vi "Encode Channels.vi"(6 "Offset":i32, 8 "error in":errorcluster, 10 "Data and Parameters":T2 {"Data" format="%.0b"}, 11 "Values in":dbl[](array[numeric])) -> (0 "error out":errorcluster, 3 "Data":u8[](array[numeric]), 4 "Number of Parameters":i32)   [LabVIEW 2020]
uses:
  <vilib>/NI/NI VeriStand Encoding and Decoding/Encoding.ctl
  b24d3698-aaae-4200-bf93-4b6af5480478.vi
  5b1080be-549e-4688-aad8-fb955257d8ef.vi
  b24d3698-aaae-4200-bf93-4b6af5480478.vi/9377bb8f-44b5-4a8f-87f1-966fd5a9edcc.vi
  b24d3698-aaae-4200-bf93-4b6af5480478.vi/e95d9d1f-307c-44d6-9f26-c3f519a4990d.vi
  b24d3698-aaae-4200-bf93-4b6af5480478.vi/0c23f515-4369-4514-bc3d-4444e6b437b2.vi
  5b1080be-549e-4688-aad8-fb955257d8ef.vi/136dcdcb-2dd3-4a4d-a796-a8f7a3f8e1ac.vi
  5b1080be-549e-4688-aad8-fb955257d8ef.vi/a54b505c-1216-4ef4-8378-3ceda9d188df.vi
  <vilib>/NI/NI VeriStand Encoding and Decoding/Get Bits Per Digit from Base.vi
  Tx UDP Execution Unit/Tx UDP Execution Unit.lvclass
  <vilib>/NI/NI VeriStand Encoding and Decoding/Encoding and Decoding.lvlib
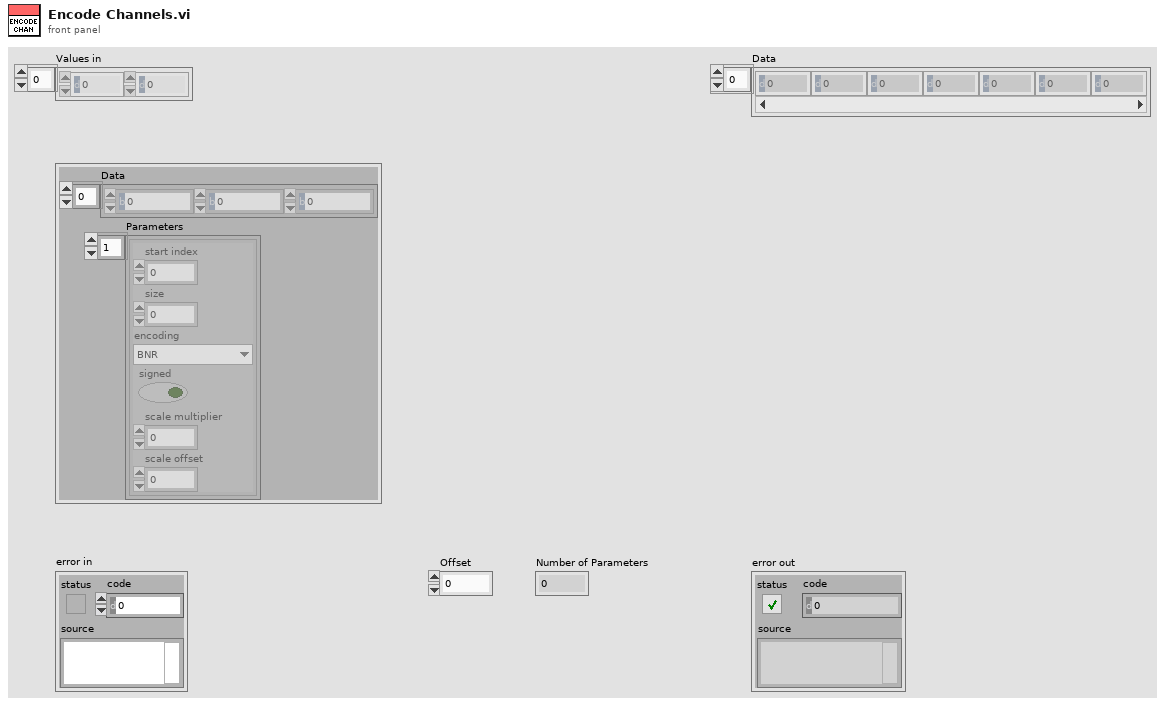
[diagram p1: front panel]
types:
  T1 = typedef "Encoding and Decoding.lvlib/Encoding.ctl" = enum16{"BNR", "BCD", "Discrete"}
  T2 = cluster{"Data":u8[], "Parameters":cluster{"start index":i32, "size":i32, "encoding":T1, "signed":bool, "scale multiplier":dbl, "scale offset":dbl}[]}
  T3 = cluster{"start index":i32, "size":i32, "encoding":T1, "signed":bool, "scale multiplier":dbl, "scale offset":dbl}[]
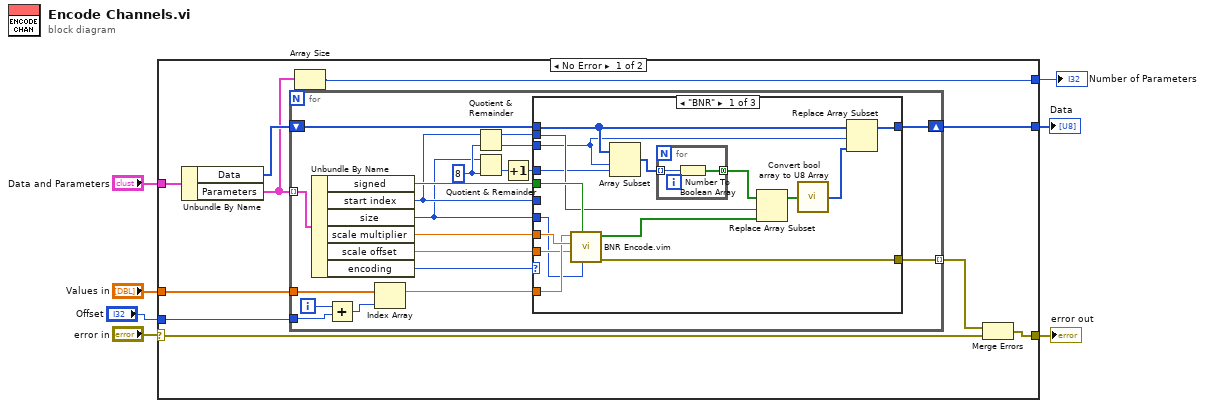
[diagram p0: block diagram]
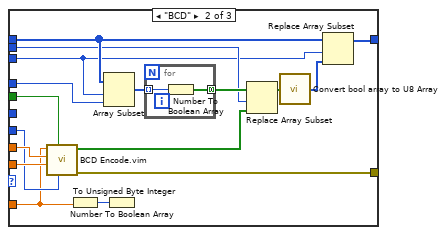
[diagram p2: hidden frame]
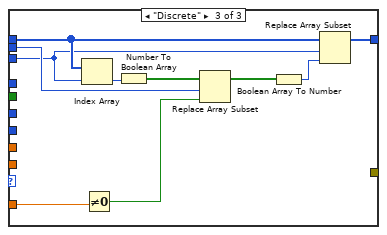
[diagram p3: hidden frame]
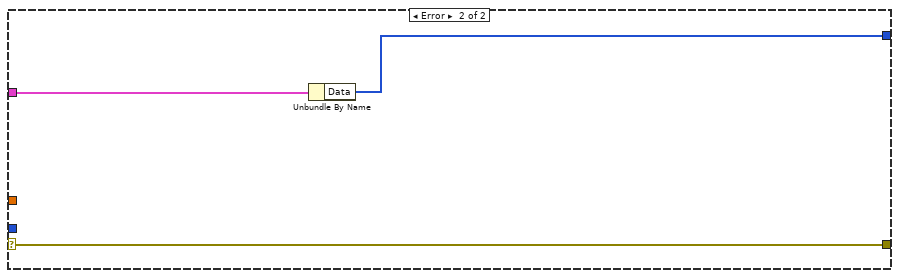
[diagram p4: hidden frame]
diagram:
  n1 = case shown="No Error" "error in" {
    selector: "error in" -> [w11 w87]
    tunnel: "Data and Parameters" -> [w17 w86]
    tunnel: "Values in" -> [w16 _]
    tunnel: [w14 w85] -> w5
    tunnel: [w12 w87] -> w3
    tunnel: "Offset" -> [w10 _]
    tunnel: [w8 _] -> w1
    frame No Error {
      n2 = Unbundle By Name(w17) -> ("Data"=w15:u8[], "Parameters"=w9:T3)
      n3 = for {
        tunnel: w16 -> [w31]
        tunnel: w9 -> [w32] mode=indexing
        shift-right: [w27] -> w14
        shift-left: w15 -> [w34]
        tunnel: [w22] -> w13 mode=indexing
        tunnel: w10 -> [w18]
        i -> [w20]
        w29 = 8 ("y")
        n4 = Unbundle By Name(w32) -> ("signed"=w33:bool, "start index"=w30:i32, "size"=w28:i32, "scale multiplier"=w36:dbl, "scale offset"=w35:dbl, "encoding"=w37:T1)
        n5 = Add(x=w20, y=w18) -> (x+y=w19:i32)
        n6 = Index Array(array=w31, index=w19) -> (element=w21:dbl)
        n7 = Quotient & Remainder(x=w30, y=w29) -> (x-y*floor(x/y)=w25:i32, floor(x/y)=w26:i32)
        n8 = Quotient & Remainder(x=w28, y=w29) -> (floor(x/y)=w24:i32)  [unwired: 1 out]
        n9 = Increment(x=w24) -> (x+1=w23:i32)
        n10 = case shown="\"BNR\"" w37 {
          tunnel: w33 -> [w53 w72 _]
          tunnel: w36 -> [w52 w71 _]
          tunnel: w35 -> [w50 w70 _]
          tunnel: w34 -> [w48 w68 w84]
          tunnel: w30 -> [_ _ _]
          tunnel: w28 -> [w49 w69 _]
          tunnel: w21 -> [w51 w60 w79]
          tunnel: [w46 w67 w83] -> w27
          tunnel: w26 -> [w38 w56 w76]
          tunnel: w25 -> [w47 w57 w80]
          tunnel: w23 -> [w43 w64 _]
          tunnel: [w39 w61 _] -> w22
          frame "BNR" {
            n11 = call "BNR Encode.vim"("data size (bits)"=w49, "signed"=w53, "scale offset"=w50, "scale multiplier"=w52, "value"=w51) -> ("error out"=w39:errorcluster, "BNR encoded value"=w42:bool[])  [unwired: 5 in]
            n12 = Array Subset(array=w48, index=w38, length=w43) -> (w45:u8[])
            n13 = for {
              tunnel: w45 -> [w55] mode=indexing
              tunnel: [w54] -> w44 mode=concatenating
              n14 = Number To Boolean Array(number=w55) -> (Boolean array=w54:bool[])
            }
            n15 = Replace Array Subset(array=w44, new element=w42, index=w47) -> (w41:bool[])
            n16 = call "Convert bool array to U8 Array.vi"("Boolean array"=w41) -> ("Array"=w40:u8[])  [unwired: 14 in]
            n17 = Replace Array Subset(array=w48, new element=w40, index=w38) -> (w46:u8[])
          }
          frame "BCD" {
            n18 = call "BCD Encode.vim"("data size (bits)"=w69, "signed"=w72, "scale offset"=w70, "scale multiplier"=w71, "value"=w60) -> ("error out"=w61:errorcluster, "BCD encoded value"=w58:bool[])  [unwired: 4 in, 1 out]
            n19 = To Unsigned Byte Integer(number=w60) -> (unsigned 8bit integer=w59:u8)
            n20 = Array Subset(array=w68, index=w56, length=w64) -> (w66:u8[])
            n21 = Number To Boolean Array(number=w59) -> ()  [unwired: 1 out]
            n22 = for {
              tunnel: w66 -> [w74] mode=indexing
              tunnel: [w73] -> w65 mode=concatenating
              n23 = Number To Boolean Array(number=w74) -> (Boolean array=w73:bool[])
            }
            n24 = Replace Array Subset(array=w65, new element=w58, index=w57) -> (w63:bool[])
            n25 = call "Convert bool array to U8 Array.vi"("Boolean array"=w63) -> ("Array"=w62:u8[])  [unwired: 14 in]
            n26 = Replace Array Subset(array=w68, new element=w62, index=w56) -> (w67:u8[])
          }
          frame "Discrete" {
            n27 = Index Array(array=w84, index=w76) -> (element=w82:u8)
            n28 = Not Equal To 0?(x=w79) -> (x != 0?=w78:bool)
            n29 = Number To Boolean Array(number=w82) -> (Boolean array=w81:bool[])
            n30 = Replace Array Subset(array=w81, new element=w78, index=w80) -> (w77:bool[])
            n31 = Boolean Array To Number(Boolean array=w77) -> (number=w75:u32)
            n32 = Replace Array Subset(array=w84, new element=w75, index=w76) -> (w83:u8[])
          }
        }
      }
      n33 = Array Size(array=w9) -> (size(s)=w8:i32)
      n34 = Merge Errors(w13, w11) -> (w12:errorcluster)
    }
    frame Error {
      n35 = Unbundle By Name(w86) -> ("Data"=w85:u8[])
    }
  }
  "Data" <- w5
  "error out" <- w3
  "Number of Parameters" <- w1
